vi "ofdm_mes_ce.vi"(11 "ZF \nchannel \nestimates":cdb[](array[numeric])) -> (0 "CSI (tx1 to rx1) 2":cdb[](array[numeric]), 1 "CSI (tx1 to rx1)":cdb[](array[numeric]), 3 "interpolated\n mes carrier CE":cdb[](array[numeric]))   [LabVIEW 2020]
panel:
  out "ZF size":i32
  out "CSI 2 size":i32
  out "CSI 1 size":i32
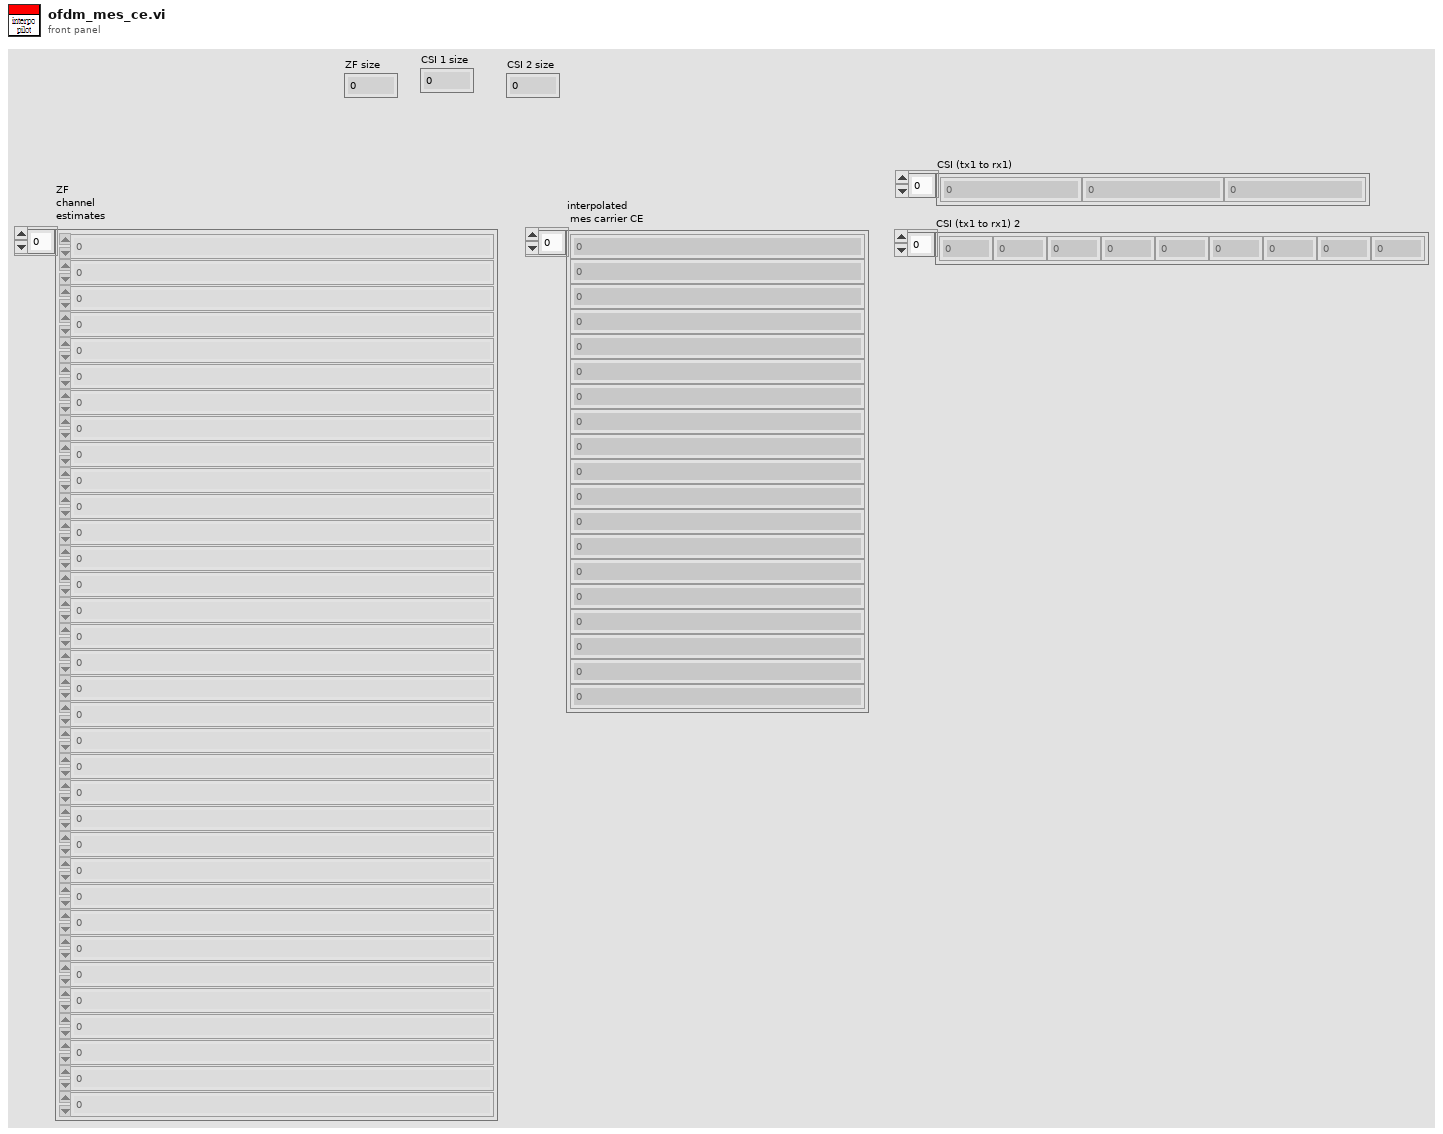
[diagram p1: front panel]
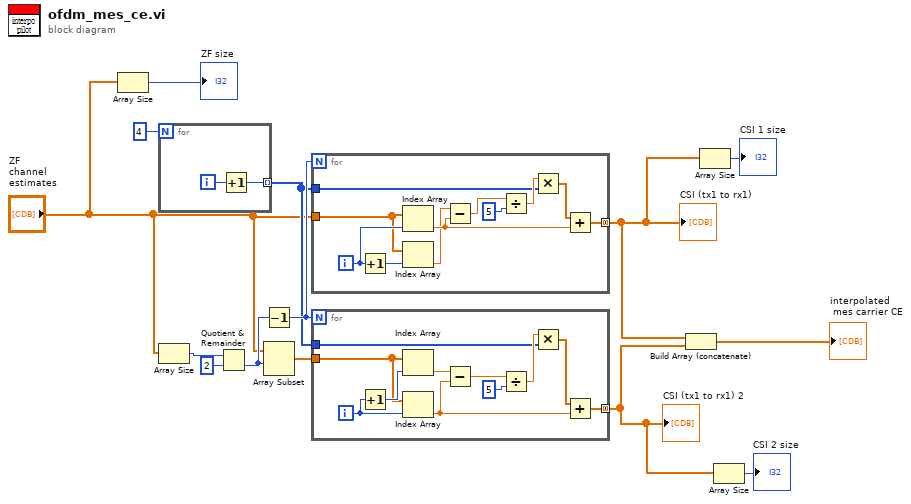
[diagram p0: block diagram]
diagram:
  n1 = Array Size(array="ZF \nchannel \nestimates") -> (size(s)=→"ZF size":i32)
  n2 = for {
    N: 4 -> [_]
    tunnel: [w15] -> w9 mode=indexing
    i -> [w16]
    n3 = Increment(x=w16) -> (x+1=w15:i32)
  }
  n4 = Array Size(array="ZF \nchannel \nestimates") -> (size(s)=w14:i32)
  n5 = Quotient & Remainder(x=w14, y=2) -> (floor(x/y)=w12:i32)  [unwired: 1 out]
  n6 = Decrement(x=w12) -> (x-1=w11:i32)
  n7 = Array Subset(array="ZF \nchannel \nestimates", index=w12) -> (w8:cdb[])  [unwired: 1 in]
  n8 = for {
    N: w11 -> [_]
    tunnel: "ZF \nchannel \nestimates" -> [w25]
    tunnel: w9 -> [w21]
    tunnel: [w19] -> w6 mode=concatenating
    i -> [w26]
    n9 = Increment(x=w26) -> (x+1=w27:i32)
    n10 = Index Array(array=w25, index=w26) -> (element=w18:cdb)
    n11 = Index Array(array=w25, index=w27) -> (element=w17:cdb)
    n12 = Subtract(x=w17, y=w18) -> (x-y=w24:cdb)
    n13 = Divide(x=w24, y=5) -> (x/y=w22:cdb)
    n14 = Multiply(x=w22, y=w21) -> (x*y=w20:cdb[])
    n15 = Add(x=w20, y=w18) -> (x+y=w19:cdb[])
  }
  "CSI (tx1 to rx1)" <- w6
  n16 = for {
    N: w11 -> [_]
    tunnel: w8 -> [w33]
    tunnel: w9 -> [w31]
    tunnel: [w30] -> w3 mode=concatenating
    i -> [w32]
    n17 = Increment(x=w32) -> (x+1=w34:i32)
    n18 = Index Array(array=w33, index=w34) -> (element=w29:cdb)
    n19 = Index Array(array=w33, index=w32) -> (element=w28:cdb)
    n20 = Subtract(x=w29, y=w28) -> (x-y=w35:cdb)
    n21 = Divide(x=w35, y=5) -> (x/y=w37:cdb)
    n22 = Multiply(x=w37, y=w31) -> (x*y=w38:cdb[])
    n23 = Add(x=w38, y=w28) -> (x+y=w30:cdb[])
  }
  "CSI (tx1 to rx1) 2" <- w3
  n24 = Build Array (concatenate) "Build Array"(w6, w3) -> (→"interpolated\n mes carrier CE":cdb[])
  n25 = Array Size(array=w6) -> (size(s)=→"CSI 1 size":i32)
  n26 = Array Size(array=w3) -> (size(s)=→"CSI 2 size":i32)
